vi "temp.vi"() -> ()   [LabVIEW 2015]
panel:
  out "Controller ID# Found":u8
  out "Encoder 2":i32
  out "Encoder 1":i32
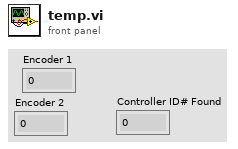
[diagram p1: front panel]
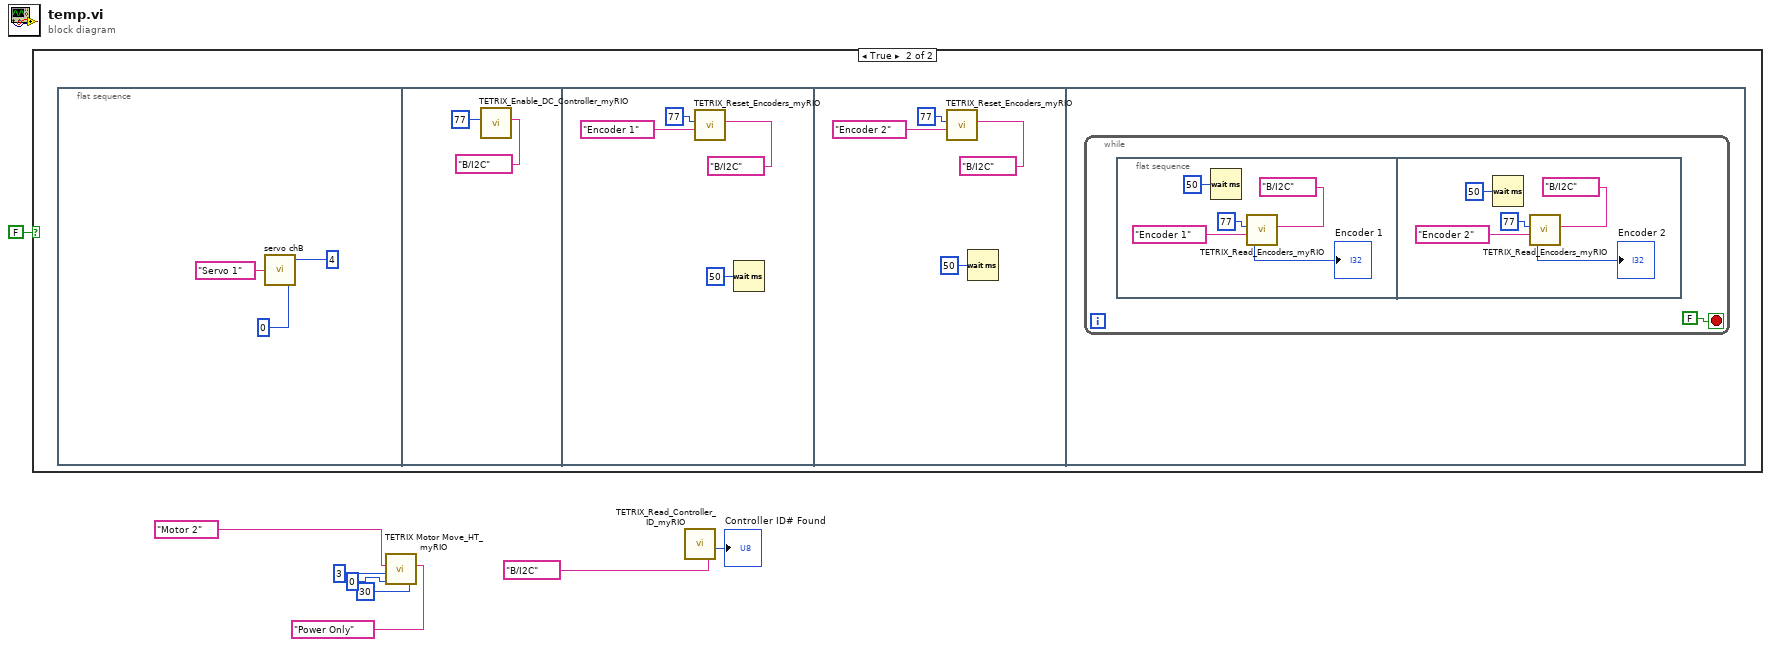
[diagram p0: block diagram]
diagram:
  n1 = case shown="True" FALSE {
    frame False {
    }
    frame True {
      n2 = flat-sequence {
        frame #0 {
          n3 = call "servo chB.vi"("Servo Position (0 - 255)"=u8 0, "Controller Daisy Chain Position (1 - 4)"=u8 4, "Select Servo"="Servo 1") -> ()  [unwired: 2 in, 1 out]
        }
        frame #1 {
          n4 = call <vilib>:"TETRIX_Enable_DC_Controller_myRIO.vi"("myRIO MXP Port A/B"=tag "B/I2C", "Controller ID#  (I2C Address)"=u8 77) -> ()  [unwired: 5 in, 1 out]
        }
        frame #2 {
          n5 = call <vilib>:"TETRIX_Reset_Encoders_myRIO.vi"("myRIO MXP Port A/B"=tag "B/I2C", "Select Encoder"="Encoder 1", "Controller ID#  (I2C Address)"=u8 77) -> ()  [unwired: 4 in, 1 out]
          n6 = Wait (ms)(milliseconds to wait=u32 50) -> ()  [unwired: 1 out]
        }
        frame #3 {
          n7 = call <vilib>:"TETRIX_Reset_Encoders_myRIO.vi"("myRIO MXP Port A/B"=tag "B/I2C", "Select Encoder"="Encoder 2", "Controller ID#  (I2C Address)"=u8 77) -> ()  [unwired: 4 in, 1 out]
          n8 = Wait (ms)(milliseconds to wait=u32 50) -> ()  [unwired: 1 out]
        }
        frame #4 {
          n9 = while {
            stop <- FALSE stop-if-true
            n10 = flat-sequence {
              frame #0 {
                n11 = Wait (ms)(milliseconds to wait=u32 50) -> ()  [unwired: 1 out]
                n12 = call <vilib>:"TETRIX_Read_Encoders_myRIO.vi"("myRIO MXP Port A/B"=tag "B/I2C", "Select Encoder"="Encoder 1", "Controller ID#  (I2C Address)"=u8 77) -> ("Encoder Output"=→"Encoder 1":i32)  [unwired: 3 in, 1 out]
              }
              frame #1 {
                n13 = Wait (ms)(milliseconds to wait=u32 50) -> ()  [unwired: 1 out]
                n14 = call <vilib>:"TETRIX_Read_Encoders_myRIO.vi"("myRIO MXP Port A/B"=tag "B/I2C", "Select Encoder"="Encoder 2", "Controller ID#  (I2C Address)"=u8 77) -> ("Encoder Output"=→"Encoder 2":i32)  [unwired: 3 in, 1 out]
              }
            }
          }
        }
      }
    }
  }
  n15 = call <vilib>:"TETRIX Motor Move_HT_myRIO.vi"("Power (-100 to 100)\n0 = Stop/Brake\n-128 = Stop/Coast"=i8 30 ("Power (-100 to 100)\n0 = Stop/Brake\n-128 = Stop/Coast"), "Control Mode"="Power Only", "Encoder Target: 360 = 1 motor shaft revolution"=0, "Controller Daisy Chain Position: 1 - 4"=u8 3, "Select Channel"="Motor 2") -> ()  [unwired: 2 in, 1 out]
  n16 = call <vilib>:"TETRIX_Read_Controller_ID_myRIO.vi"("myRIO MXP Port A/B"=tag "B/I2C") -> ("Controller ID# Found"=→"Controller ID# Found":u8)  [unwired: 5 in, 1 out]
